vi "configure.vi"(8 "error in (no error)":errorcluster, 11 "GenericPlugin in":refnum<class "FPGAWrapperAK101022Resonance.lvclass">) -> (0 "error out":errorcluster, 3 "GenericPlugin out":refnum<class "FPGAWrapperAK101022Resonance.lvclass">)   [LabVIEW 2010, in "FPGAWrapperAK101022Resonance.lvclass"]
doc: "The dynamic dispatch version of this VI loads and displays the configuration file associated with the plug-in object. The user modify and save the configuration data."
uses:
  FPGAWrapperAK101022Resonance.lvclass
  FPGAWrapperAK101022Resonance.lvclass/FPGAWrapperAK101022Resonance.ctl
panel:
  in  "ADC clock phase":i32 min=0 max=10
  in  "button:cancel":bool
  in  "button:save":bool
  in  "Invert channels (ch0/ch1)?":bool[](array[boolean])
  in  "channel offsets":u32[](array[numeric])
  # "Configure FPGAWrapperAK101022Resonance"
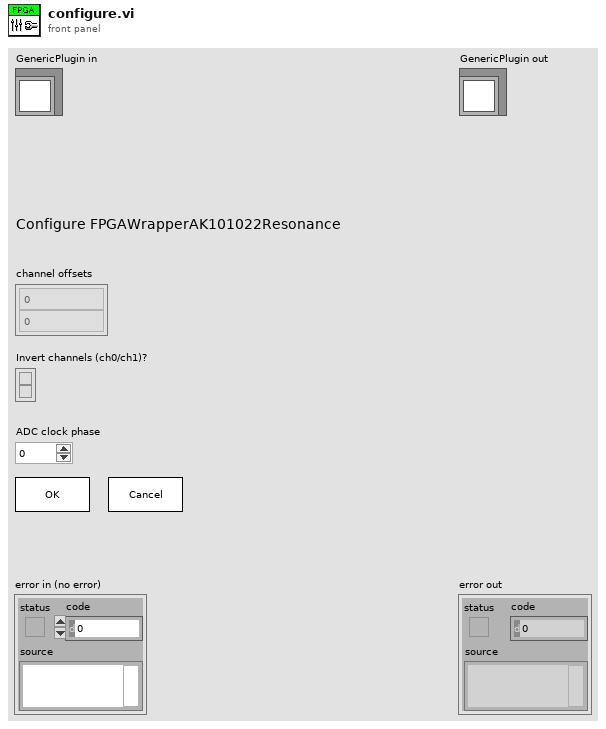
[diagram p1: front panel]
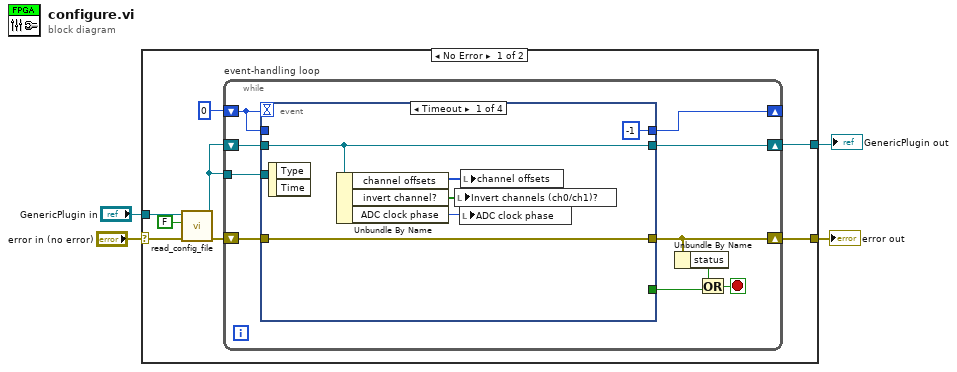
[diagram p0: block diagram]
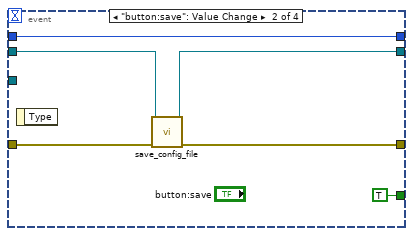
[diagram p2: hidden frame]
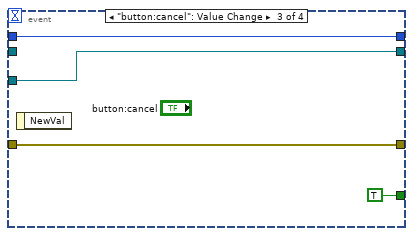
[diagram p3: hidden frame]
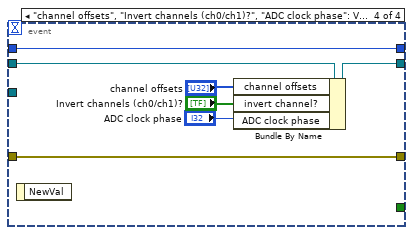
[diagram p4: hidden frame]
diagram:
  n1 = case shown="No Error" "error in (no error)" {
    selector: "error in (no error)" -> [w9 w47]
    tunnel: [w11 w47] -> w3
    tunnel: "GenericPlugin in" -> [w7 w46]
    tunnel: [w10 w46] -> w1
    frame No Error {
      n2 = call-dynamic "read_config_file.vi"("error in (no error)"=w9, "force load?"=FALSE, "GenericPlugin in"=w7) -> ("error out"=w8:errorcluster, "GenericPlugin out"=w6:refnum<class "FPGAWrapperAK101022Resonance.lvclass">)  [unwired: 7 in]
      n3 = while "event-handling loop" {
        shift-right: [w16] -> w11
        shift-left: w8 -> [w22]
        shift-right: [w20] -> _
        shift-left: 0 -> [w21]
        shift-right: [w18] -> w10
        shift-left: w6 -> [w19]
        tunnel: w6 -> [w17]
        stop <- w13 stop-if-true
        n4 = event shown="[0] Timeout" {
          selector: _ -> [_ _ _ _]
          dyn-events: _ -> [_ _ _ _]
          timeout: w21 -> [_ _ _ _]
          tunnel: w22 -> [w28 w31 w38 w45]
          tunnel: [w28 w30 w38 w45] -> w16
          tunnel: w21 -> [_ w34 w37 w44]
          tunnel: [-1 w34 w37 w44] -> w20
          tunnel: w19 -> [w26 w33 _ w41]
          tunnel: [w26 w32 w36 w40] -> w18
          tunnel: w17 -> [_ _ w36 _]
          tunnel: [_ TRUE TRUE _] -> w15
          event Timeout {
            n5 = event-data() -> ()  [unwired: 1 in, 2 out]
            n6 = Unbundle By Name(w26) -> ("channel offsets"=w25:u32[], "invert channel?"=w24:bool[], "ADC clock phase"=w23:i32)
            n7 = local write "Invert channels (ch0/ch1)?"(w24) -> ()
            n8 = local write "ADC clock phase"(w23) -> ()
            n9 = local write "channel offsets"(w25) -> ()
          }
          event "button:save": Value Change {
            n10 = event-data() -> ()  [unwired: 1 in, 1 out]
            n11 = call-dynamic "save_config_file.vi"("error in (no error)"=w31, "GenericPlugin in"=w33) -> ("error out"=w30:errorcluster, "GenericPlugin out"=w32:refnum<class "FPGAWrapperAK101022Resonance.lvclass">)  [unwired: 8 in]
          }
          event "button:cancel": Value Change {
            n12 = event-data() -> ()  [unwired: 1 in, 1 out]
          }
          event "channel offsets", "Invert channels (ch0/ch1)?", "ADC clock phase": Value Change {
            n13 = event-data() -> ()  [unwired: 1 in, 1 out]
            n14 = Bundle By Name(cluster=w41, "channel offsets"="channel offsets", "invert channel?"="Invert channels (ch0/ch1)?", "ADC clock phase"="ADC clock phase") -> (w40:refnum<class "FPGAWrapperAK101022Resonance.lvclass">)
          }
        }
        n15 = Unbundle By Name(w16) -> ("status"=w14:bool)
        n16 = Or(x=w14, y=w15) -> (x .or. y?=w13:bool)
      }
    }
    frame Error {
    }
  }
  "error out" <- w3
  "GenericPlugin out" <- w1
